vi "Preview AI Channel.vi"(7 "index":i32, 8 "error in":errorcluster, 10 "samples":u32=2048, 11 "host in":refnum<class "LIA Host Interface FPGA.lvclass">) -> (0 "error out":errorcluster, 2 "samples out":i16[](array[numeric]), 3 "host out":refnum<class "LIA Host Interface FPGA.lvclass">)   [LabVIEW 2017, in "LIA Host Interface FPGA.lvclass"]
uses:
  LIA Host Interface FPGA.lvclass
  Properties/FpgaSession_GET.vi
  host/Lock-In Amplifier Example Host.lvlib
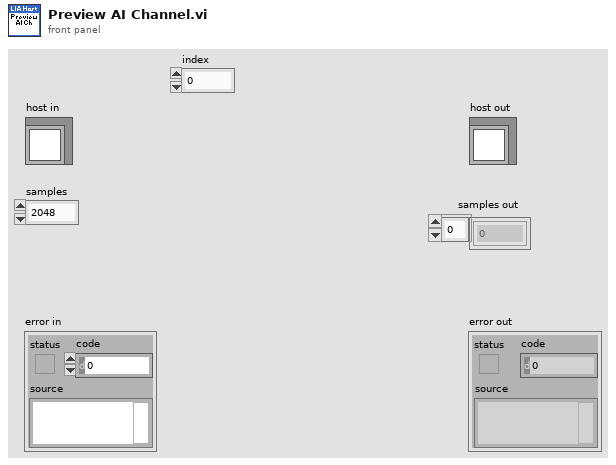
[diagram p1: front panel]
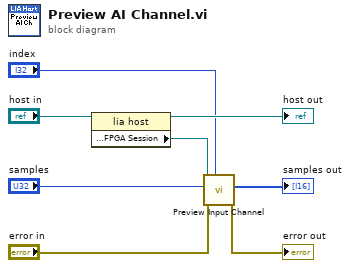
[diagram p0: block diagram]
diagram:
  n1 = property class="lia host"(reference="host in") -> (reference out=→"host out":refnum<class "LIA Host Interface FPGA.lvclass">, "Properties:FPGA Session"=w6:refnum<k20>)  [unwired: 1 in, 1 out]
  n2 = call "Preview Input Channel.vi"("channel"="index", "error in"="error in", "samples"="samples", "fpga session in"=w6) -> ("error out"=→"error out":errorcluster, "ai data"=→"samples out":i16[])  [unwired: 5 in, 1 out]
